vi "RunMeas.vi"(8 "error in (no error)":errorcluster, 11 "ChromaPowerSupply in":refnum<class "ChromaPowerSupply.lvclass">) -> (0 "error out":errorcluster, 2 "variant":variant, 3 "ChromaPowerSupply out":refnum<class "ChromaPowerSupply.lvclass">)   [LabVIEW 2018, in "AcPwrPlugins.lvlib" / "ChromaPowerSupply.lvclass"]
doc: "This VI initiates and takes measurements from the instrument(s)."
uses:
  ChromaPowerSupply.lvclass
  AcPwrShared/clMeasurmentData.ctl
  AcPwrShared/clAcPwrAttributes.ctl
  AcPwrShared/AcPwrShared.lvlib
  ChromaAcLoadClass/ChromaAcLoad.lvclass
panel:
  in  "Measure Type (Voltage)":i32(ring) items=["Voltage", "Current", "Power"]
  out "Waveform Chart":waveform(dbl)[](graph)
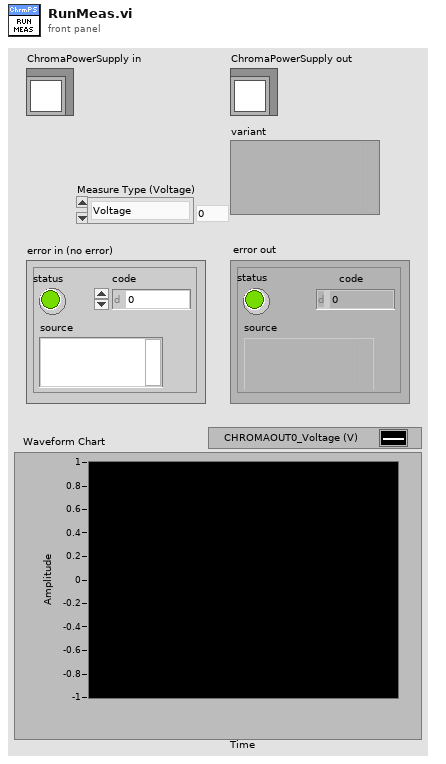
[diagram p1: front panel]
types:
  T1 = typedef "AcPwrPlugins.lvlib/ChromaPowerSupply.lvclass/Measurements.ctl" = cluster{"Handle":string, "Name":string, "Enabled":bool, "Measurement Value":dbl, "btnMeasFetch":bool, "ProtectionStatusString":string, "Measurement Type":enum16{"Voltage", "Current", "Power"}}[]
  T2 = typedef "AcPwrPlugins.lvlib/ChromaPowerSupply.lvclass/Device(s)Settings.ctl" = cluster{"Phases":cluster{"Handle":string, "Instrument Options":string, "id query (T)":bool, "reset device (T)":bool, "Timing":cluster{"TimingOn":enum16{""}, "Hours":u32, "Minutes":u32, "Seconds":dbl, "CutoffVoltage":dbl}, "Connected":bool, "Output Mode":enum16{"Voltage (DC)", "Current (DC)"}, "Voltage":dbl, "Current":dbl, "High Voltage Limit":dbl, "High Current Limit":dbl, "Power Protect":dbl, "Current Protect":dbl, "Voltage Protect":dbl, "Low Current Limit":dbl, "Low Voltage Limit":dbl, "Current Slew Rate":dbl, "Voltage Slew Rate":dbl, "Current Slew Infinite?":bool}[], "MeasName":string}
  T3 = typedef "AcPwrShared.lvlib/clMeasurmentData.ctl" = cluster{"MeasName":string, "XML Data":string, "WaveformData":waveform(dbl)[]}
  T4 = typedef "AcPwrShared.lvlib/clAcPwrAttributes.ctl" = cluster{"ProtectionStatusString":string, "Handle_MeasurementType":string, "Status Byte Register":cluster{"Busy":bool, "Remote Mode":bool, "Error in Queue":bool, "QUES=Questionable Status Summary":bool, "MAV = Message Available":bool, "ESB = Event Status Byte Summary":bool, "RQS = Request for Service":bool, "OPER = Operation Event Summary":bool}}
  T5 = cluster{"Handle":string, "Name":string, "Enabled":bool, "Measurement Value":dbl, "btnMeasFetch":bool, "ProtectionStatusString":string, "Measurement Type":enum16{"Voltage", "Current", "Power"}}
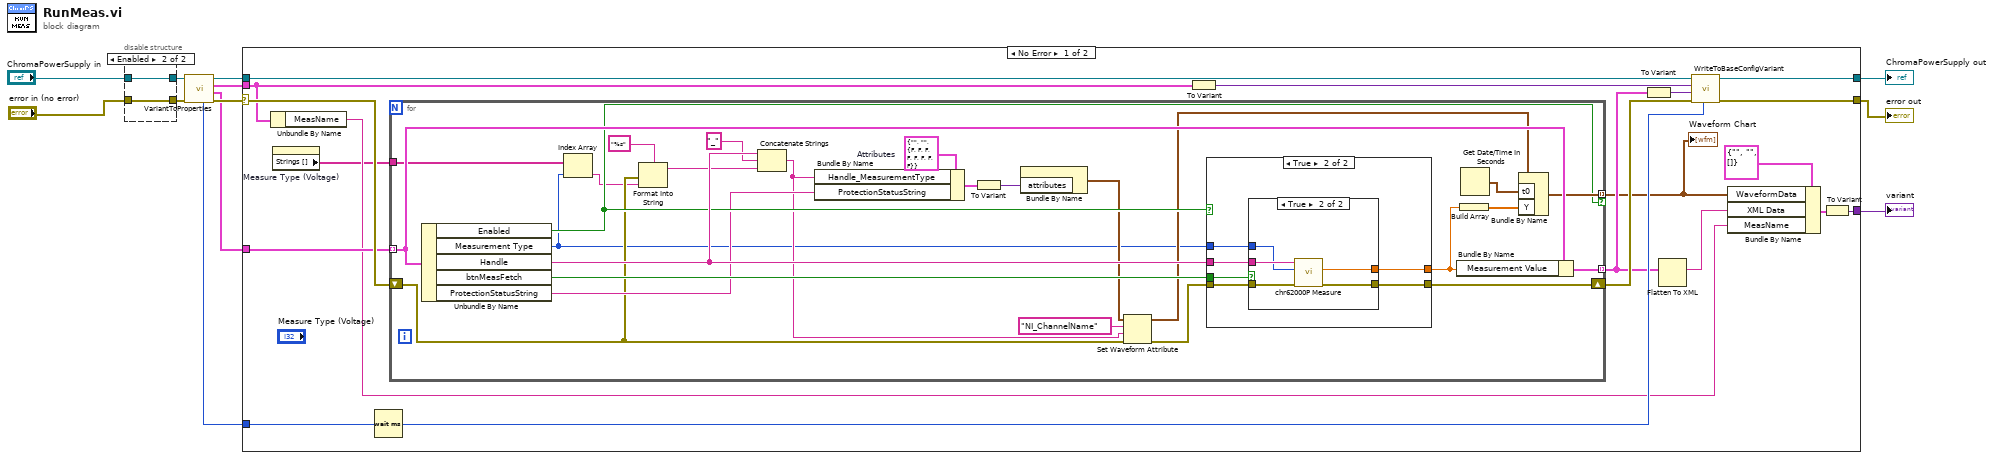
[diagram p0: block diagram]
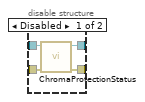
[diagram p2: hidden frame]
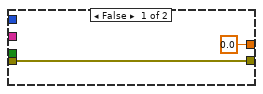
[diagram p3: hidden frame]
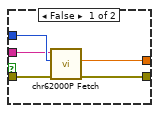
[diagram p4: hidden frame]
diagram:
  n1 = disable-structure shown="Enabled" {
    disable-tunnel: [w16 w17] -> w12
    disable-tunnel: [w15 w18] -> w11
    disable-tunnel: "ChromaPowerSupply in" -> [w14 w18]
    disable-tunnel: "error in (no error)" -> [w13 w17]
    frame Disabled {
      n2 = call "ChromaProtectionStatus.vi"("error in (no error)"=w13, "ChromaAcLoad in"=w14) -> ("error out"=w16:errorcluster, "ChromaAcLoad out"=w15:refnum<class "ChromaAcLoad.lvclass">)  [unwired: 8 in]
    }
    frame Enabled {
    }
  }
  n3 = call-dynamic "VariantToProperties.vi"("error in (no error)"=w12, "ChromaPowerSupply in"=w11) -> ("error out"=w7:errorcluster, "Measurements"=w6:T1, "Device Settings"=w5:T2, "ChromaPowerSupply out"=w9:refnum<class "ChromaPowerSupply.lvclass">, "Measurement Refresh Time (ms)"=w4:u32)  [unwired: 5 in]
  n4 = case shown="No Error" w7 {
    selector: w7 -> [w37 w82]
    tunnel: [w33 w83] -> w3
    tunnel: [w31 w82] -> w1
    tunnel: w9 -> [w35 w83]
    tunnel: w5 -> [w28 _]
    tunnel: w6 -> [w36 _]
    tunnel: w4 -> [w29 _]
    tunnel: [w21 _] -> w2
    frame No Error {
      n5 = Unbundle By Name(w28) -> ("MeasName"=w22:string)
      n6 = property on="Measure Type (Voltage)" class="Ring (strict)"() -> ("Strings []"=w19:string[])  [unwired: 2 in, 2 out]
      n7 = Wait (ms)(milliseconds to wait=w29) -> (millisecond timer value=w27:u32)
      n8 = for {
        tunnel: w36 -> [w63] mode=indexing
        shift-right: [w61] -> w34
        shift-left: w37 -> [w41]
        tunnel: [w62] -> w26 mode=indexing
        tunnel: [w57] -> w20 mode=indexing if=w50
        tunnel: w19 -> [w40]
        w49 = T4 {"ProtectionStatusString"="", "Handle_MeasurementType"="", "Status Byte Register"={"Busy"=FALSE, "Remote Mode"=FALSE, "Error in Queue"=FALSE, "QUES=Questionable Status Summary"=FALSE, "MAV = Message Available"=FALSE, "ESB = Event Status Byte Summary"=FALSE, "RQS = Request for Service"=FALSE, "OPER = Operation Event Summary"=FALSE}}  # Attributes
        n9 = Unbundle By Name(w63) -> ("Enabled"=w50:bool, "Measurement Type"=w39:enum16{"Voltage", "Current", "Power"}, "Handle"=w53:string, "btnMeasFetch"=w60:bool, "ProtectionStatusString"=w47:string)
        n10 = Index Array(array=w40, index=w39) -> (element=w38:string)
        n11 = Format Into String(format string="%s", error in=w41, w38) -> (resulting string=w51:string)  [unwired: 1 in, 1 out]
        n12 = Concatenate Strings(w53, "_", w51) -> (w43:string)
        n13 = Bundle By Name(cluster=w49, "Handle_MeasurementType"=w43, "ProtectionStatusString"=w47) -> (w48:T4)
        n14 = To Variant(anything=w48) -> (Variant=w54:variant)
        n15 = Bundle By Name("attributes"=w54) -> (w42:waveform(dbl))  [unwired: 1 in]
        n16 = Set Waveform Attribute(4:w41, 5:w43, 6:"NI_ChannelName" ("name"), 7:w42) -> (0:w45:errorcluster, 3:w44:waveform(dbl))  [unwired: 1 out]
        n17 = case shown="True" w50 {
          tunnel: w45 -> [w65 w68]
          tunnel: w39 -> [_ w67]
          tunnel: [w65 w69] -> w61
          tunnel: [0.0 ("Query CF of Current") w66] -> w59
          tunnel: w53 -> [_ w70]
          tunnel: w60 -> [_ w71]
          frame False {
          }
          frame True {
            n18 = case shown="True" w71 {
              tunnel: w70 -> [w74 w81]
              tunnel: [w73 w80] -> w69
              tunnel: w68 -> [w76 w79]
              tunnel: w67 -> [w75 w77]
              tunnel: [w72 w78] -> w66
              frame False {
                n19 = call <instrlib>:"chr62000P Fetch.vi"("error in (no error)"=w76, "Fetch Type (Voltage)"=w75, "instrument handle"=w74) -> ("error out"=w73:errorcluster, "ReadValue"=w72:dbl)  [unwired: 6 in, 1 out]
              }
              frame True {
                n20 = call <instrlib>:"chr62000P Measure.vi"("error in (no error)"=w79, "Measure Type (Voltage)"=w77, "instrument handle"=w81) -> ("error out"=w80:errorcluster, "ReadValue"=w78:dbl)  [unwired: 6 in, 1 out]
              }
            }
          }
        }
        n21 = Bundle By Name(cluster=w63, "Measurement Value"=w59) -> (w62:T5)
        n22 = Build Array(w59) -> (w58:dbl[])
        n23 = Get Date/Time In Seconds() -> (seconds since 1Jan1904=w56:timestamp)
        n24 = Bundle By Name(cluster=w44, "t0"=w56, "Y"=w58) -> (w57:waveform(dbl))
      }
      "Waveform Chart" <- w20
      n25 = To Variant(anything=w28) -> (Variant=w30:variant)
      n26 = To Variant(anything=w26) -> (Variant=w32:variant)
      n27 = Flatten To XML(anything=w26) -> (xml string=w23:string)
      n28 = call-dynamic "WriteToBaseConfigVariant.vi"("Measurement Refresh Time (ms)"=w27, "error in (no error)"=w34, "Meas"=w32, "Config"=w30, "ChromaPowerSupply in"=w35) -> ("error out"=w31:errorcluster, "ChromaPowerSupply out"=w33:refnum<class "ChromaPowerSupply.lvclass">)  [unwired: 5 in]
      n29 = Bundle By Name(cluster=T3 {"MeasName"="", "XML Data"="", "WaveformData"=[]} ("MeasurmentDataCluster"), "WaveformData"=w20, "XML Data"=w23, "MeasName"=w22) -> (w24:T3)
      n30 = To Variant(anything=w24) -> (Variant=w21:variant)
    }
    frame Error {
    }
  }
  "ChromaPowerSupply out" <- w3
  "error out" <- w1
  "variant" <- w2
